vi "velocity.vi"() -> (3 "v[km/h]":dbl)   [LabVIEW 2015]
uses:
  G_VEH.vi
  G_PATH.vi
panel:
  out "output variable":dbl
  out "subarray":dbl[](array[numeric])
  out "d":dbl
  out "vr":dbl
  out "va":dbl
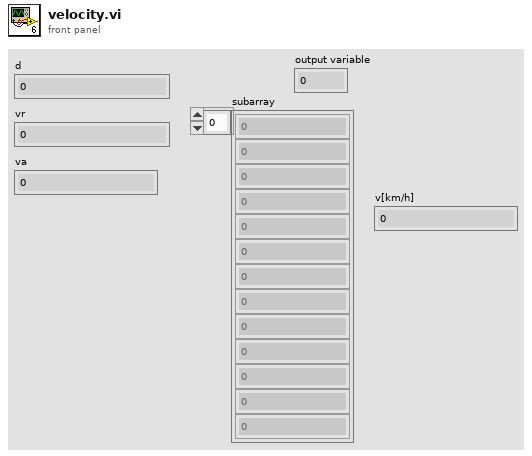
[diagram p1: front panel]
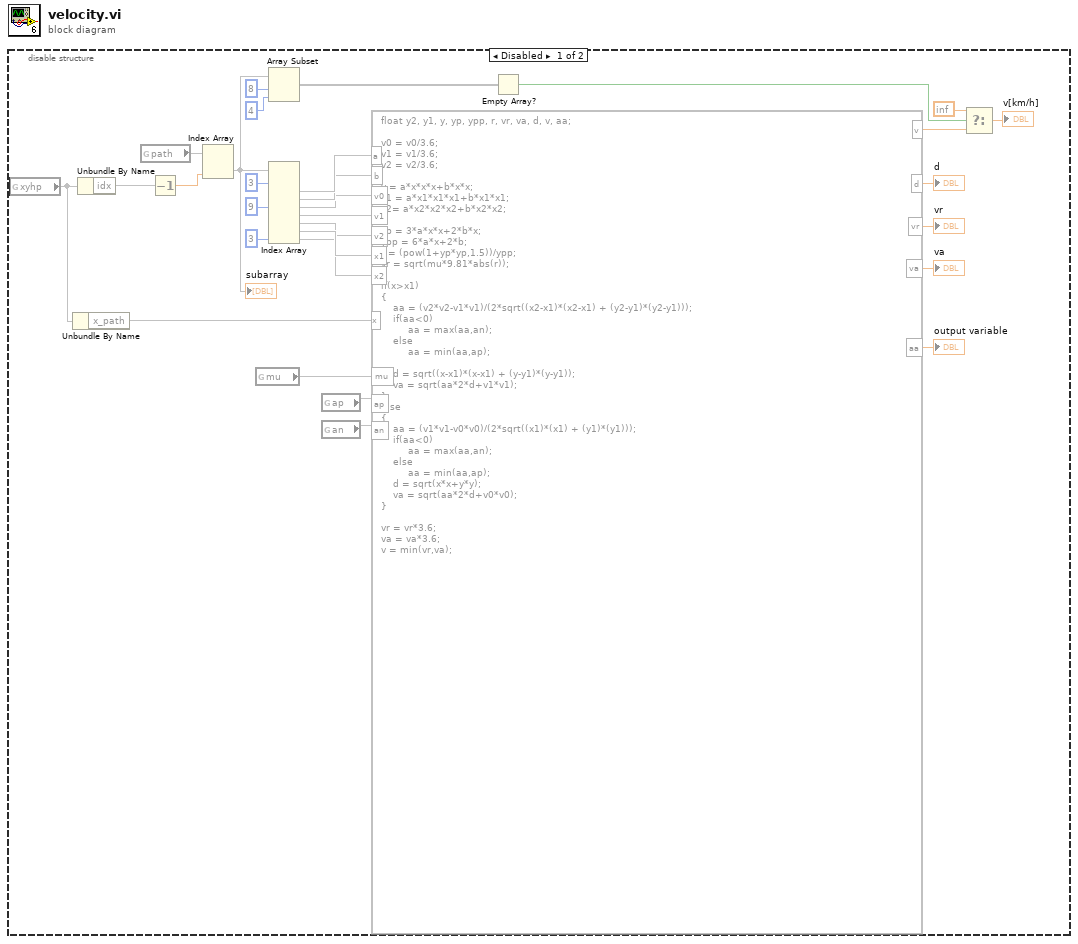
[diagram p0: block diagram]
diagram:
  n1 = disable-structure shown="Disabled" {
    frame Disabled {
      n2 = global read "G_VEH.vi" "xyhp"() -> (w10)
      n3 = Unbundle By Name(w10) -> ("x_path"=w21)
      n4 = Unbundle By Name(w10) -> ("idx"=w30)
      n5 = global read "G_PATH.vi" "path"() -> (w1)
      n6 = Decrement(x=w30) -> (x-1=w29:dbl)
      n7 = Index Array(array=w1, index (col)=w29) -> (element=w9)  [unwired: 1 in]
      "subarray" <- w9
      n8 = global read "G_VEH.vi" "mu"() -> (w11)
      n9 = Array Subset(array=w9, index=8, length=4) -> (w6:void[])
      n10 = Index Array(array=w9, index #1=3 ("index"), index #4=9 ("index"), index #8=3 ("index")) -> (element #2=w28, element #3=w27, element #4=w24, element #5=w23, element #6=w14, element #7=w22, element #8=w16)  [unwired: 5 in, 1 out]
      n11 = global read "G_VEH.vi" "ap"() -> (w12)
      n12 = global read "G_VEH.vi" "an"() -> (w13)
      n13 = formula code="float y2, y1, y, yp, ypp, r, vr, va, d, v, aa;\n\nv0 = v0/3.6;\nv1 = v1/3.6;\nv2 = v2/3.6;\n\ny = a*x*x*x+b*x*x;\ny1 = a*x1*x1*x1+b*x1*x1;\ny2= a*x2*x2*x2+b*x2*x2;\n\nyp = 3*a*x*x+2*b*x;\nypp = 6*a*x+2*b;\nr = (pow(1+yp*yp,1.5))/ypp;\nvr = sqrt(mu*9.81*abs(r));\n\nif(x>x1)\n{        \n    aa = (v2*v2-v1*v1)/(2*sqrt((x2-x1)*(x2-x1) + (y2-y1)*(y2-y1)));\n    if(aa<0)\n         aa = max(aa,an);\n    else\n         aa = min(aa,ap);\n\n    d = sqrt((x-x1)*(x-x1) + (y-y1)*(y-y1));\n    va = sqrt(aa*2*d+v1*v1);\n}\nelse\n{\n    aa = (v1*v1-v0*v0)/(2*sqrt((x1)*(x1) + (y1)*(y1)));\n    if(aa<0)\n         aa = max(aa,an);\n    else\n         aa = min(aa,ap);\n    d = sqrt(x*x+y*y);\n    va = sqrt(aa*2*d+v0*v0);\n}\n\nvr = vr*3.6;\nva = va*3.6;\nv = min(vr,va);"("a"=w28, "b"=w27, "x"=w21, "mu"=w11, "v0"=w24, "v1"=w23, "v2"=w14, "x1"=w22, "ap"=w12, "an"=w13, "x2"=w16) -> ("v"=w3:dbl, "d"=→"d":dbl, "vr"=→"vr":dbl, "va"=→"va":dbl, "aa"=→"output variable":dbl)
      n14 = Empty Array?(array=w6) -> (empty?=w5:bool)
      n15 = Select(t=inf, s=w5, f=w3) -> (s? t:f=→"v[km/h]":dbl)
    }
    frame Enabled {
    }
  }
